vi "Sound File to Sound Output.vi"() -> ()   [LabVIEW 2014]
doc: "This VI illustrates how to play a sound file continuously, reading the sound file in pieces, and playing each piece at a time."
uses:
  <vilib>/sound2/lvsound2.llb/Sampling Mode.ctl
  <vilib>/sound2/lvsound2.llb/Sound File Info (path).vi
  <vilib>/sound2/lvsound2.llb/Sound File Read Open.vi
  <vilib>/sound2/lvsound2.llb/Sound File Read (DBL).vi
  <vilib>/sound2/lvsound2.llb/Sound Output Write (DBL).vi
panel:
  out "Current Data":waveform(dbl)[](graph)
  out "Current Iteration":i32
  in  "Stop":bool
  in  "Number of Samples/Iteration":i32=2500
  in  "Device ID":u32
  # "Overview: Demonstrates the use of the Sound VIs to play a sound file continuously, reading the sound file in pieces, and playing each piece one at a time.\nInstructions:\n1. Specify the Device ID and the Number of Samples/Iteration.\n2. Run the VI."
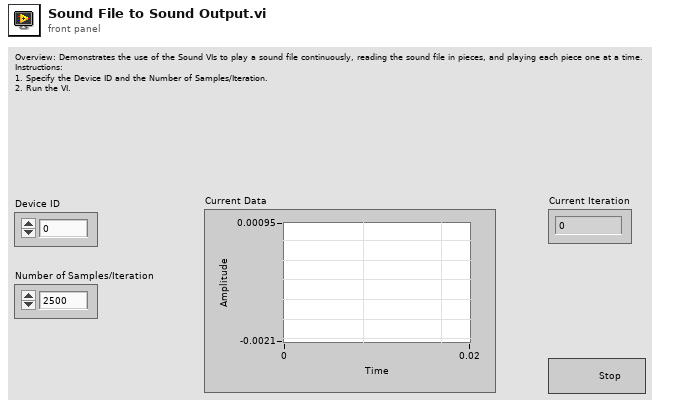
[diagram p1: front panel]
types:
  T1 = typedef "Sampling Mode.ctl" = i32
  T2 = typedef "Sound Data Format.ctl" = cluster{"sample rate (S/s)":dbl, "number of channels":i32, "bits per sample":i32}
  T3 = typedef "Sound File Refnum.ctl" = refnum<file>
  T4 = typedef "Sound Output Task ID.ctl" = u32
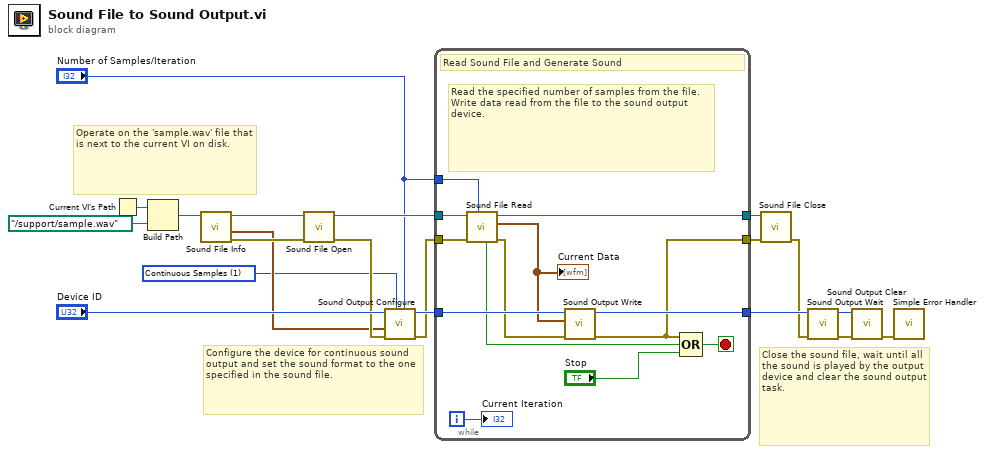
[diagram p0: block diagram]
diagram:
  w5 = T1 1 items=["Finite Samples", "Continuous Samples"] ("sample mode")
  # "Operate on the 'sample.wav' file that is next to the current VI on disk."
  # "Close the sound file, wait until all the sound is played by the output device and clear the sound output task."
  # "Configure the device for continuous sound output and set the sound format to the one specified in the sound file."
  n1 = Current VI's Path() -> (path=w1:path)
  n2 = Build Path(base path=w1, name or relative path=path "../support/sample.wav" ("Sound File Path")) -> (appended path=w2:path)
  n3 = call-poly <vilib>:"Sound File Info.vi"("path"=w2) -> ("error out"=w15:errorcluster, "sound format"=w7:T2, "path out"=w8:path)  [unwired: 7 in, 1 out]
  n4 = call-poly <vilib>:"Sound File Open.vi"("error in (no error)"=w15, "path"=w8) -> ("error out"=w14:errorcluster, "sound file refnum"=w16:T3)  [unwired: 8 in]
  n5 = call <vilib>:"Sound Output Configure.vi"("number of samples/ch"="Number of Samples/Iteration", "sample mode"=w5, "error in (no error)"=w14, "sound format"=w7, "device ID"="Device ID") -> ("error out"=w13:errorcluster, "task ID"=w20:T4)  [unwired: 5 in]
  n6 = while {
    tunnel: "Number of Samples/Iteration" -> [w23]
    tunnel: w16 -> [w31]
    tunnel: [w29] -> w18
    tunnel: w13 -> [w32]
    tunnel: [w22] -> w17
    tunnel: w20 -> [w28]
    tunnel: [w33] -> w11
    i -> [w30]
    stop <- w24 stop-if-true
    # "Read the specified number of samples from the file. Write data read from the file to the sound output device."
    # "Read Sound File and Generate Sound"
    n7 = call-poly <vilib>:"Sound File Read.vi"("number of samples/ch (-1: all)"=w23, "error in (no error)"=w32, "sound file refnum"=w31) -> ("error out"=w27:errorcluster, "data"=w21:waveform(dbl)[], "sound file refnum out"=w29:T3, "end of file?"=w25:bool)  [unwired: 4 in, 1 out]
    "Current Data" <- w21
    n8 = call-poly <vilib>:"Sound Output Write.vi"("error in (no error)"=w27, "data"=w21, "task ID"=w28) -> ("error out"=w22:errorcluster, "task ID out"=w33:T4)  [unwired: 7 in]
    n9 = Compound Arithmetic op=OR(w22, w25, "Stop") -> (w24:bool)
    "Current Iteration" <- w30
  }
  n10 = call <vilib>:"Sound File Close.vi"("error in (no error)"=w17, "sound file refnum"=w18) -> ("error out"=w10:errorcluster)  [unwired: 9 in]
  n11 = call <vilib>:"Sound Output Wait.vi"("error in (no error)"=w10, "task ID"=w11) -> ("error out"=w9:errorcluster, "task ID out"=w12:T4)  [unwired: 8 in]
  n12 = call <vilib>:"Sound Output Clear.vi"("error in (no error)"=w9, "task ID"=w12) -> ("error out"=w4:errorcluster)  [unwired: 9 in]
  n13 = call <vilib>:"Simple Error Handler.vi"("error in (no error)"=w4) -> ()  [unwired: 4 in, 5 out]
